vi "OAT Analog Tacho Process.vi"   [LabVIEW 2017, in "SoundVib_TachProcess.lvlib"]
doc: "Locates tachometer pulse positions in analog tachometer signals using the number of generated pulses per revolution, the pulse width, and the arrival edge of the tachometer pulse. This VI also calculates the rotational speed of the device. Wire data to the <B>analog tacho signal</B> input to determine the polymorphic instance to use or manually select the instance."
uses:
  <vilib>/addons/Sound and Vibration/Order Analysis/Tach Process/SoundVib_TachProcess.lvlib
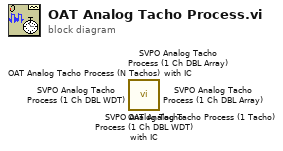
[diagram p0: block diagram]
diagram:
  n1 = call <vilib>:"SVPO Analog Tacho Process (1 Ch DBL WDT) with IC.vi"() -> ()  [unwired: 13 in, 3 out]
  n2 = call <vilib>:"SVPO Analog Tacho Process (1 Ch DBL Array) with IC.vi"() -> ()  [unwired: 13 in, 3 out]
  n3 = call <vilib>:"SVPO Analog Tacho Process (1 Ch DBL WDT).vi"() -> ()  [unwired: 14 in, 2 out]
  n4 = call <vilib>:"SVPO Analog Tacho Process (1 Ch DBL Array).vi"() -> ()  [unwired: 14 in, 2 out]
  n5 = call <vilib>:"OAT Analog Tacho Process (N Tachos).vi"() -> ()  [unwired: 11 in, 5 out]
  n6 = call <vilib>:"OAT Analog Tacho Process (1 Tacho).vi"() -> ()  [unwired: 11 in, 5 out]
